vi "trace_mean.vi"(8 "Reset":bool=TRUE, 11 "Array in":sgl[][][](array[numeric])) -> (3 "Array out":sgl[][](array[numeric]))   [LabVIEW 2013]
uses:
  probe_point.ctl
  <vilib>/Analysis/4window.llb/Hanning Window (DBL).vi
  <vilib>/Analysis/4window.llb/AllCosWindow (DBL).vi
  <vilib>/Analysis/NI_AALPro.lvlib
panel:
  # "Decimate of a block of trace data records, OR'ing flags.   We apply a window  as a low-order decimation filter."
  # "If true, this is the first (or only) point in a time series."
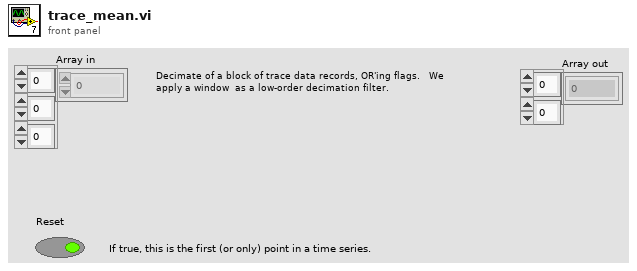
[diagram p1: front panel]
types:
  T1 = typedef "probe_point.ctl" = enum16{"Position (tip)", "Position (RCM)", "Null pos (tip)", "Null pos (RCM)", "V limiter (tip)", "V Limiter (RCM)", "Goal (tip)", "Goal (RCM)", "Link pos 0", "Link pos 1", "KF link pos 0", "KF link pos 1", "Link rate 0", "Link rate 1", "Link residue 0", "Link residue 1", "Link goal 0", "Link goal 1", "Rate limit 0", "Rate limit 1", "Link error 0", "Link error 1", "Controller 0", "Controller 1", "Output 0", "Output 1", "Drive 0", "Drive 1", "Stimulus 0", "Stimulus 1", "Trace data 0", "Trace data 1", "Analog data 0", "Analog data 1", "Status flags", "Light 0", "Light 1", "Light 2", "Light 3", "Light 4", "Light 5", "Goal origin", "Goal rotation 0", "Goal rotation 1", "Goal rotation 2", "Output origin", "Output rotation 0", "Output rotation 1", "Output rotation 2", "Handle origin", "Handle rotation 0", "Handle rotation 1", "Handle rotation 2", "Handle position", "Handle velocity", "Handle acceleration", "Handle angles", "Handle angle rates", "Handle pos residue", "Handle angle residue", "Trace length"}
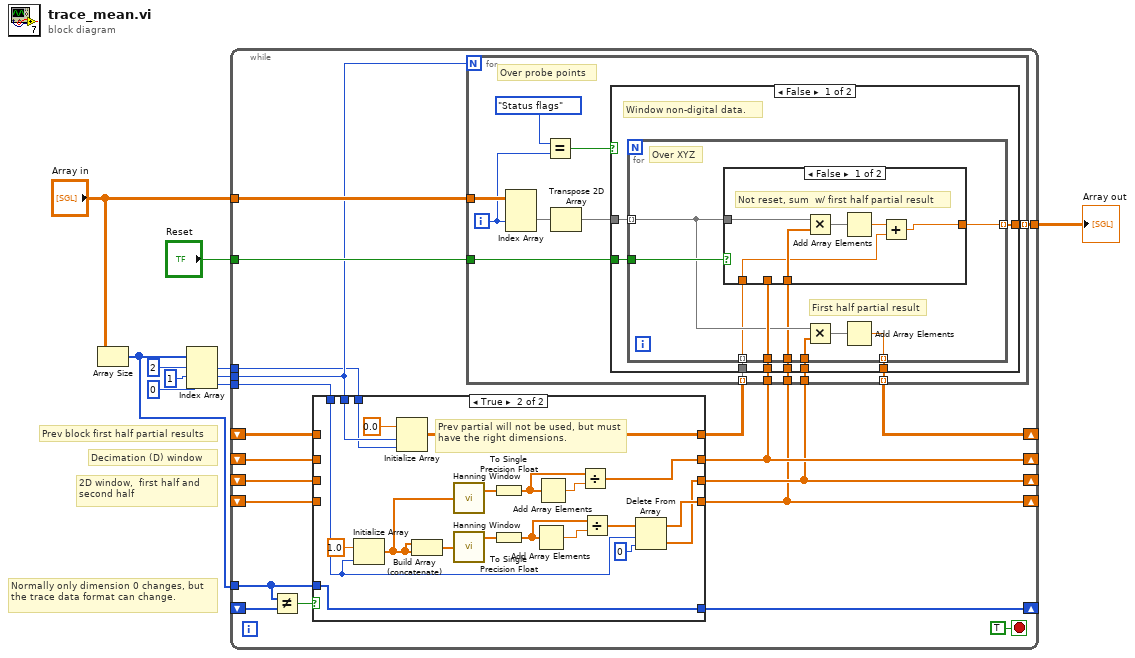
[diagram p0: block diagram]
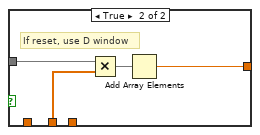
[diagram p3: hidden frame]
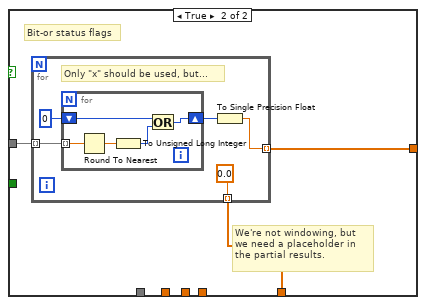
[diagram p4: hidden frame]
diagram:
  # "Normally only dimension 0 changes, but the trace data format can change."
  # "2D window,  first half and \nsecond half"
  # "Decimation (D) window"
  # "Prev block first half partial results"
  n1 = Array Size(array="Array in") -> (size(s)=w1:i32[])
  n2 = Index Array(array=w1, index #1=2 ("index"), index #2=1 ("index"), index #3=0 ("index")) -> (element #1=w2:i32, element #2=w8:i32, element #3=w6:i32)
  n3 = while {
    tunnel: "Array in" -> [w30]
    tunnel: [w29] -> w9
    tunnel: w8 -> [w14]
    tunnel: w6 -> [w24]
    shift-right: [w25] -> _
    shift-left: _ -> [w27]
    shift-right: [w18] -> _
    shift-left: _ -> [w22]
    shift-right: [w19] -> _
    shift-left: _ -> [w23]
    shift-right: [w17] -> _
    shift-left: _ -> [w15]
    shift-right: [w16] -> _
    shift-left: _ -> [w21]
    tunnel: "Reset" -> [w20]
    tunnel: w2 -> [w13]
    tunnel: w1 -> [w11]
    stop <- TRUE stop-if-true
    n4 = Not Equal?(x=w11, y=w27) -> (x != y?=w26:bool)
    n5 = case shown="True" w26 {
      tunnel: [w31 w37] -> w25
      tunnel: w24 -> [_ w36]
      tunnel: [w35 w46] -> w19
      tunnel: [w33 w49] -> w16
      tunnel: [w34 w48] -> w18
      tunnel: w23 -> [w35 _]
      tunnel: w22 -> [w34 _]
      tunnel: w21 -> [w33 _]
      tunnel: w15 -> [w32 _]
      tunnel: w14 -> [_ w40]
      tunnel: w13 -> [_ w39]
      tunnel: [w32 w38] -> w12
      tunnel: w11 -> [w31 w37]
      frame False {
      }
      frame True {
        # "Prev partial will not be used, but must have the right dimensions."
        n6 = Initialize Array(1.0 ("element"), w36) -> (w54:dbl[])
        n7 = Initialize Array(sgl 0.0 ("sum"), w40, w39) -> (w38:sgl[][])
        n8 = Build Array (concatenate)(w54, w54) -> (w53:dbl[])
        n9 = call-poly <vilib>:"Hanning Window.vi"("X"=w54) -> ("Windowed X"=w52:dbl[])  [unwired: 1 out]
        n10 = call-poly <vilib>:"Hanning Window.vi"("X"=w53) -> ("Windowed X"=w51:dbl[])  [unwired: 1 out]
        n11 = To Single Precision Float(number=w52) -> (single precision float=w47:sgl[])
        n12 = To Single Precision Float(number=w51) -> (single precision float=w43:sgl[])
        n13 = Add Array Elements(numeric array=w43) -> (sum=w44:sgl)
        n14 = Add Array Elements(numeric array=w47) -> (sum=w45:sgl)
        n15 = Divide(x=w47, y=w45) -> (x/y=w46:sgl[])
        n16 = Divide(x=w43, y=w44) -> (x/y=w42:sgl[])
        n17 = Delete From Array(array=w42, length=w36, index=0) -> (deleted portion=w48:sgl[], array with subset deleted=w49:sgl[])
      }
    }
    n18 = for {
      N: w14 -> [_]
      tunnel: w30 -> [w68]
      tunnel: [w65] -> w29 mode=indexing
      tunnel: w20 -> [w61]
      tunnel: w19 -> [w60]
      tunnel: w18 -> [w59]
      tunnel: [w58] -> w17 mode=indexing
      tunnel: w12 -> [w57] mode=indexing
      tunnel: w16 -> [w56]
      i -> [w63]
      # "Over probe points"
      n19 = Index Array(array=w68, index (dim 1)=w63) -> (element=w67:sgl[][])  [unwired: 2 in]
      n20 = Equal?(x=probe_point."Status flags" ("Probe point"), y=w63) -> (x = y?=w62:bool)
      n21 = Transpose 2D Array(2D array=w67) -> (transposed array=w66:sgl[][])
      n22 = case shown="False" w62 {
        tunnel: w66 -> [w76 w98]
        tunnel: [w73 w97] -> w65
        tunnel: w61 -> [w75 _]
        tunnel: w60 -> [w74 _]
        tunnel: w59 -> [w72 _]
        tunnel: [w71 w96] -> w58
        tunnel: w57 -> [w70 _]
        tunnel: w56 -> [w69 _]
        frame False {
          # "Window non-digital data."
          n23 = for {
            tunnel: w76 -> [w81] mode=indexing
            tunnel: w75 -> [w85]
            tunnel: w74 -> [w84]
            tunnel: [w83] -> w73 mode=indexing
            tunnel: w72 -> [w80]
            tunnel: [w79] -> w71 mode=indexing
            tunnel: w70 -> [w78] mode=indexing
            tunnel: w69 -> [w77]
            # "First half partial result"
            # "Over XYZ"
            n24 = case shown="False" w85 {
              tunnel: w81 -> [w91 w95]
              tunnel: w84 -> [_ w93]
              tunnel: [w86 w92] -> w83
              tunnel: w78 -> [w88 _]
              tunnel: w77 -> [w89 _]
              frame False {
                # "Not reset, sum  w/ first half partial result"
                n25 = Multiply(x=w91, y=w89) -> (x*y=w90:sgl[])
                n26 = Add Array Elements(numeric array=w90) -> (sum=w87:sgl)
                n27 = Add(x=w87, y=w88) -> (x+y=w86:sgl)
              }
              frame True {
                # "If reset, use D window"
                n28 = Multiply(x=w95, y=w93) -> (x*y=w94:sgl[])
                n29 = Add Array Elements(numeric array=w94) -> (sum=w92:sgl)
              }
            }
            n30 = Multiply(x=w81, y=w80) -> (x*y=w82:sgl[])
            n31 = Add Array Elements(numeric array=w82) -> (sum=w79:sgl)
          }
        }
        frame True {
          # "We're not windowing, but\nwe need a placeholder in\nthe partial results."
          # "Bit-or status flags"
          n32 = for {
            tunnel: w98 -> [w101] mode=indexing
            tunnel: [w100] -> w97 mode=indexing
            tunnel: [sgl 0.0 ("single precision float")] -> w96 mode=indexing
            # "Only \"x\" should be used, but..."
            n33 = for {
              shift-right: [w106] -> w102
              shift-left: u16 0 ("unsigned 16bit integer") -> [w107]
              tunnel: w101 -> [w104] mode=indexing
              n34 = Round To Nearest(number=w104) -> (nearest integer value=w105:sgl)
              n35 = To Unsigned Long Integer(number=w105) -> (unsigned 32bit integer=w108:u32)
              n36 = Or(x=w107, y=w108) -> (x .or. y?=w106:u32)
            }
            n37 = To Single Precision Float(number=w102) -> (single precision float=w100:sgl)
          }
        }
      }
    }
  }
  "Array out" <- w9
